vi "Logger.SearchForNewFiles.vi"(8 "error in":errorcluster) -> (0 "error out":errorcluster)   [LabVIEW 2016]
uses:
  Logger.FileBody.ctl
  Global/ApplicationGlobal.vi
panel:
  out "HandledFileContent":T1[](array[typedef]) {"Values" format="%.3f"}
  out "HandledFileContent":T1 {"Values" format="%.3f"}
  out "Array":string[](array[string])
  out "text":string
  in  "ResultsFile":u32[](array[numeric])
  out "SerialNo":string
  out "Variant":string
  out "System":string
  out "filenames":string[](array[string])
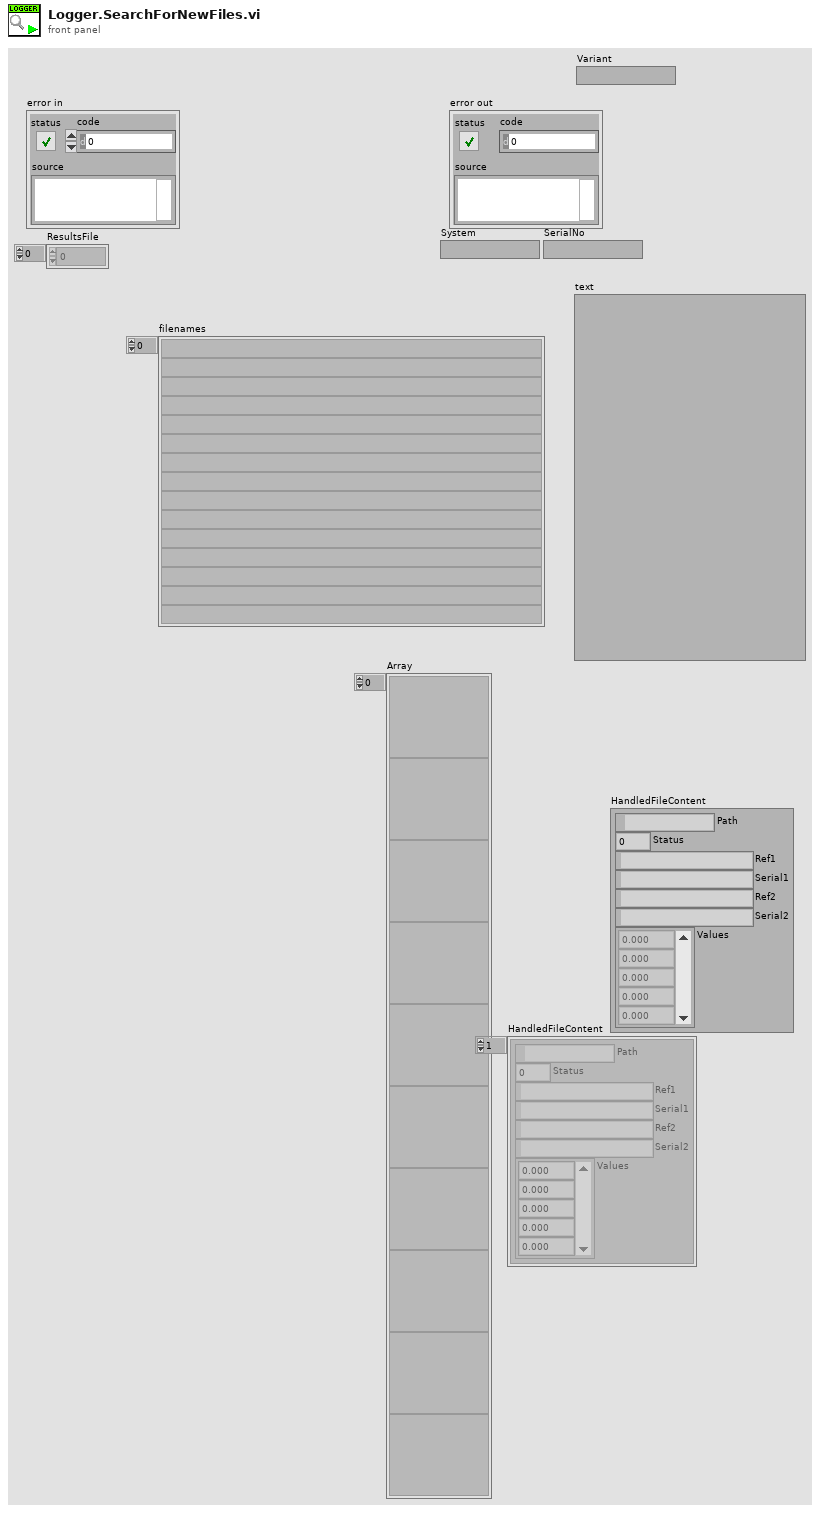
[diagram p1: front panel]
types:
  T1 = typedef "Logger.FileBody.ctl" = cluster{"Path":path, "Status":u8, "Ref1":string, "Serial1":string, "Ref2":string, "Serial2":string, "Values":sgl[]}
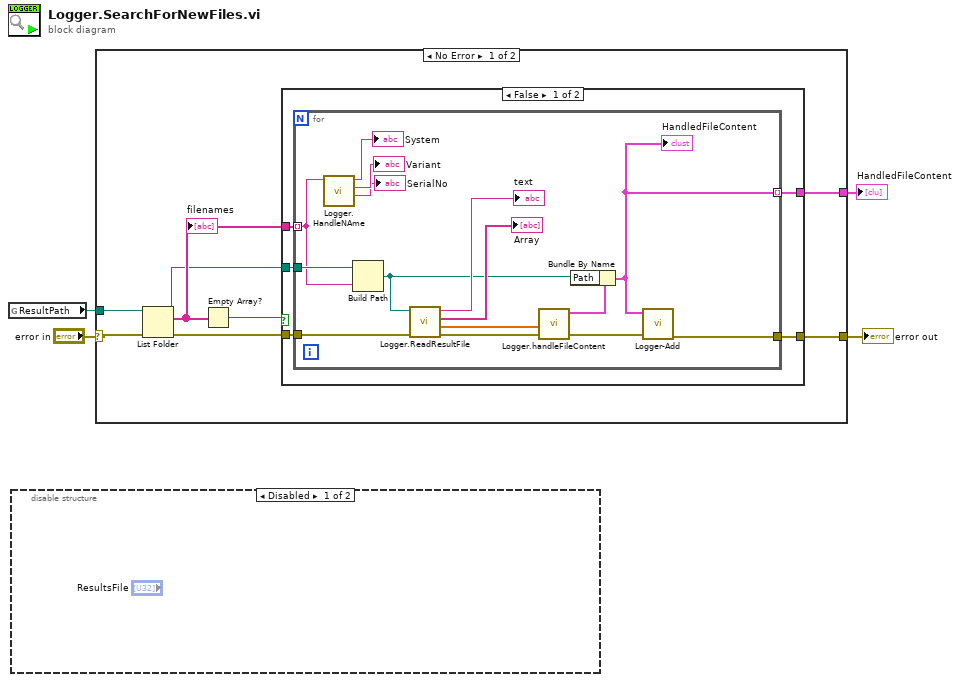
[diagram p0: block diagram]
diagram:
  n1 = global read "ApplicationGlobal.vi" "ResultPath"() -> (w2:path)
  n2 = disable-structure shown="Disabled" {
    frame Disabled {
    }
    frame Enabled {
    }
  }
  n3 = case shown="No Error" "error in" {
    selector: "error in" -> [w11 w33]
    tunnel: [w5 w33] -> w4
    tunnel: w2 -> [w12 _]
    tunnel: [w7 _] -> w1
    frame No Error {
      n4 = List Folder(path=w12, error in=w11) -> (path out=w8:path, filenames=w9:string[], error out=w6:errorcluster)  [unwired: 2 in, 1 out]
      "filenames" <- w9
      n5 = Empty Array?(array=w9) -> (empty?=w10:bool)
      n6 = case shown="False" w10 {
        tunnel: w9 -> [w17 _]
        tunnel: w8 -> [w16 _]
        tunnel: [w15 _] -> w7
        tunnel: w6 -> [w14 w32]
        tunnel: [w13 w32] -> w5
        frame False {
          n7 = for {
            tunnel: w17 -> [w27] mode=indexing
            tunnel: w16 -> [w28]
            tunnel: [w19] -> w15 mode=indexing
            tunnel: w14 -> [w23]
            tunnel: [w21] -> w13
            n8 = call "Logger.HandleNAme.vi"("String"=w27) -> ("SerialNo"=→"SerialNo":string, "Variant"=→"Variant":string, "System"=→"System":string)  [unwired: 8 in]
            n9 = Build Path(base path=w28, name or relative path=w27) -> (appended path=w18:path)
            n10 = call "Logger.ReadResultFile.vi"("error in"=w23, "ResultFilePath"=w18) -> ("error out"=w22:errorcluster, 1:"ResultValues"=w26:dbl[], 2:"ResultValues"=→"Array":string[], "text"=→"text":string)  [unwired: 6 in]
            n11 = call "Logger.handleFileContent.vi"("ResultsFile"=w26) -> ("HandledFileContent"=w20:T1)  [unwired: 10 in]
            n12 = Bundle By Name(cluster=w20, "Path"=w18) -> (w19:T1)
            "HandledFileContent" <- w19
            n13 = call "Logger-Add.vi"("error in"=w22, "HandledFileContent"=w19) -> ("error out"=w21:errorcluster)  [unwired: 9 in]
          }
        }
        frame True {
        }
      }
    }
    frame Error {
    }
  }
  "error out" <- w4
  "HandledFileContent" <- w1
